vi "Draw Target.vi"(1 "Color":u32(colorbox)=16448250, 2 "Original Image":T1(plugin-control)) -> (0 "Image Out":T1(plugin-control))   [LabVIEW 2011]
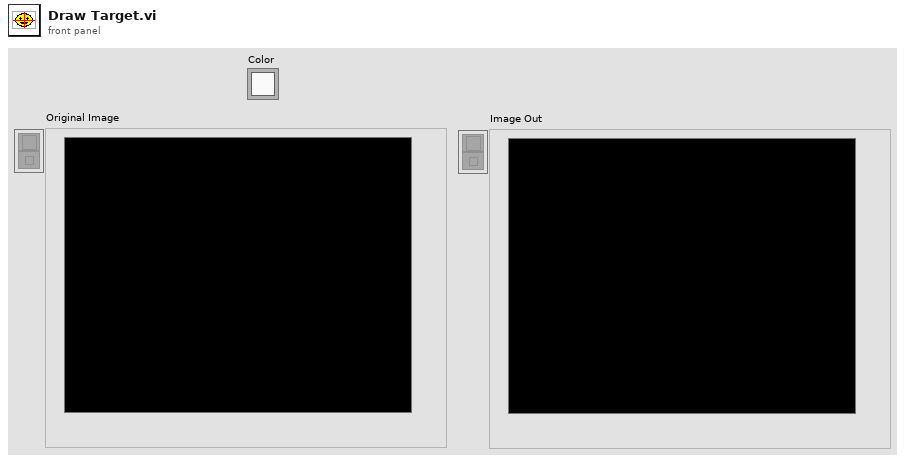
[diagram p1: front panel]
types:
  T1 = typedef "IMAQ Image.ctl" = refnum<image>
  T2 = cluster{"Left":i32, "Top":i32, "Right":i32, "Bottom":i32}
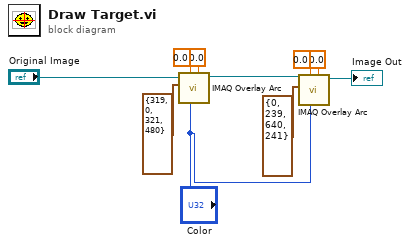
[diagram p0: block diagram]
diagram:
  n1 = call "IMAQ Overlay Arc"("End Angle (degrees)"=0.0, "Color"="Color", "Start Angle (degrees)"=0.0, "Bounding Rectangle"=T2 {"Left"=319, "Top"=0, "Right"=321, "Bottom"=480}, "Image"="Original Image") -> ("Image Out"=w3:T1)  [unwired: 5 in, 1 out]
  n2 = call "IMAQ Overlay Arc"("End Angle (degrees)"=0.0, "Color"="Color", "Start Angle (degrees)"=0.0, "Bounding Rectangle"=T2 {"Left"=0, "Top"=239, "Right"=640, "Bottom"=241}, "Image"=w3) -> ("Image Out"=→"Image Out":T1)  [unwired: 5 in, 1 out]
